vi "_Parse ES Flatness Segment Subcarrier Index Result.vi"(8 "error in (no error)":errorcluster, 10 "Input String":string, 11 "VISA resource name":refnum<visa-resource-name>) -> (0 "error out":errorcluster, 1 "Subcarrier Index Results":T2, 2 "Reliability Results":T1, 3 "VISA resource name out":refnum<visa-resource-name>, 5 "Out Of Tolerance":dbl format="%^.3e", 7 "Statistic Expired":i32)   [LabVIEW 2020, in "Rohde&Schwarz CMXP NR FR2 Measurement.lvlib"]
uses:
  <instrlib>/Rohde&Schwarz CMXP NR FR2 Measurement/Rohde&Schwarz CMXP NR FR2 Measurement.lvlib
  <instrlib>/Rohde&Schwarz CMXP NR FR2 Measurement/Private/rsidr_core.llb/rsidr_core.lvlib
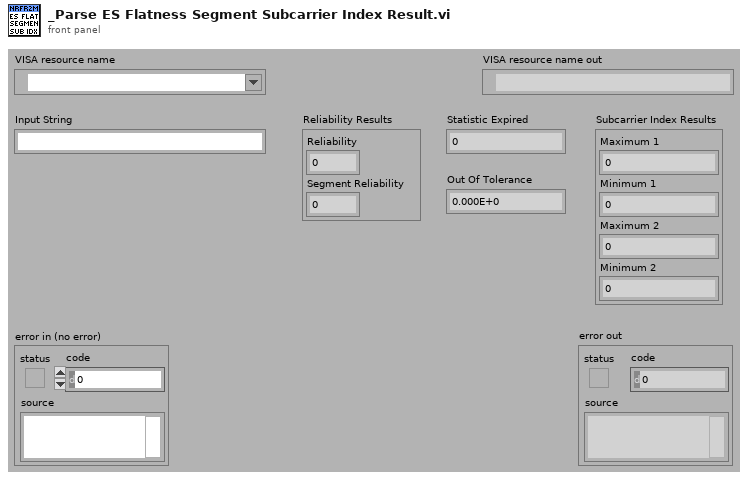
[diagram p1: front panel]
types:
  T1 = cluster{"Reliability":i32, "Segment Reliability":i32}
  T2 = cluster{"Maximum 1":i32, "Minimum 1":i32, "Maximum 2":i32, "Minimum 2":i32}
  T3 = cluster{"int32 array out[0]":i32, "int32 array out[1]":i32, "int32 array out[2]":i32, "int32 array out[3]":i32}
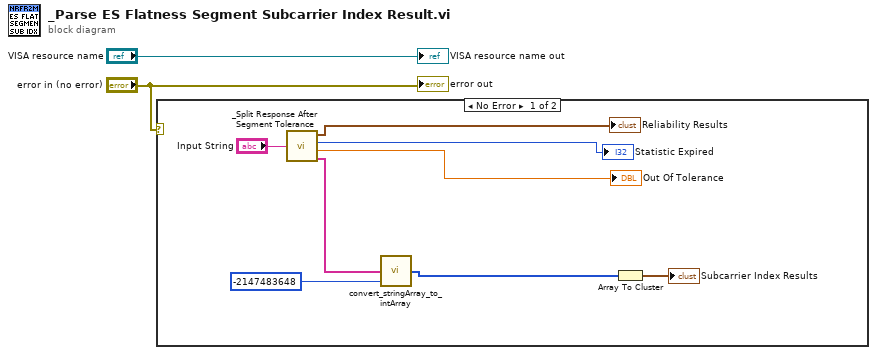
[diagram p0: block diagram]
diagram:
  n1 = case shown="No Error" "error in (no error)" {
    frame No Error {
      n2 = call <instrlib>:"_Split Response After Segment Tolerance.vi"("Input String"="Input String") -> ("Reliability Results"=→"Reliability Results":T1, "Statistic Expired"=→"Statistic Expired":i32, "Out Of Tolerance"=→"Out Of Tolerance":dbl, "Response out"=w6:string[])
      n3 = call <instrlib>:"convert_stringArray_to_intArray.vi"("default (0)"=-2147483648, "string array in"=w6) -> ("int32 array out"=w5:i32[])  [unwired: 3 in]
      n4 = Array To Cluster(array=w5) -> (cluster=→"Subcarrier Index Results":T3)
    }
    frame Error {
    }
  }
  "VISA resource name out" <- "VISA resource name"
  "error out" <- "error in (no error)"
